vi "PMTreadgraph.vi"(8 "error in":errorcluster, 10 "queue in":refnum<queue>, 11 "PMT chart":refnum<vi>) -> (0 "error out":errorcluster)   [LabVIEW 2019]
uses:
  <vilib>/Analysis/baseanly.llb/Mean (DBL).vi
  <vilib>/Utility/error.llb/Error Cluster From Error Code.vi
  <vilib>/rvi/errors/niLvFpgaAdjustHostInterfaceError.vi
  GlobalImagingStatus.vi
  <vilib>/rvi/interface/nirviReadWriteControl/nirviReadWriteControl.xnode
  <vilib>/Analysis/NI_AALBase.lvlib
  Global.lvlib
  NiFpgaLv.dll
  <vilib>/rvi/interface/Simulation/niFpgaSimulationCallBeginRW.vi
panel:
  out "PMT saturation 2":bool
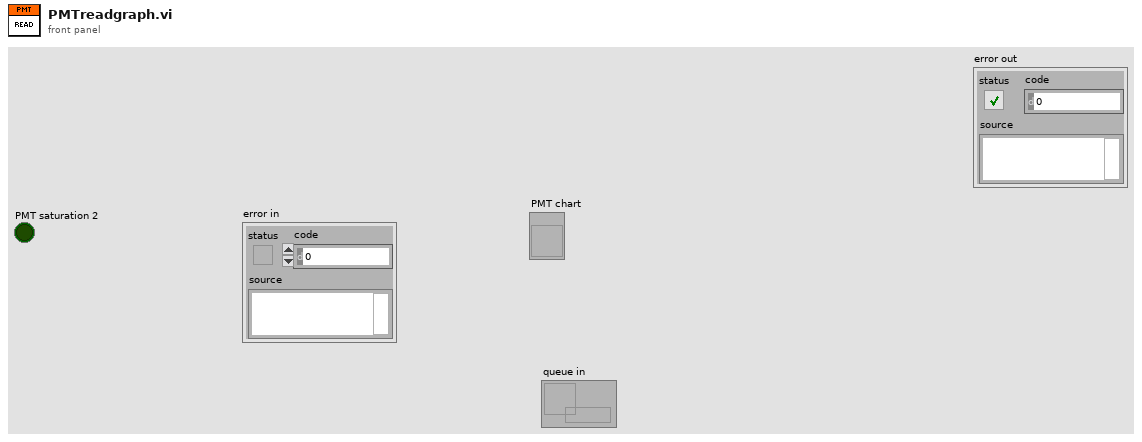
[diagram p1: front panel]
types:
  T1 = typedef "ImagingStatusControl.ctl" = enum16{"PMT_large", "Camera_large", "PMT", "Camera", "Idle"}
  T2 = cluster{"Frequency Chart":u32, "Frequency Chart":u32}
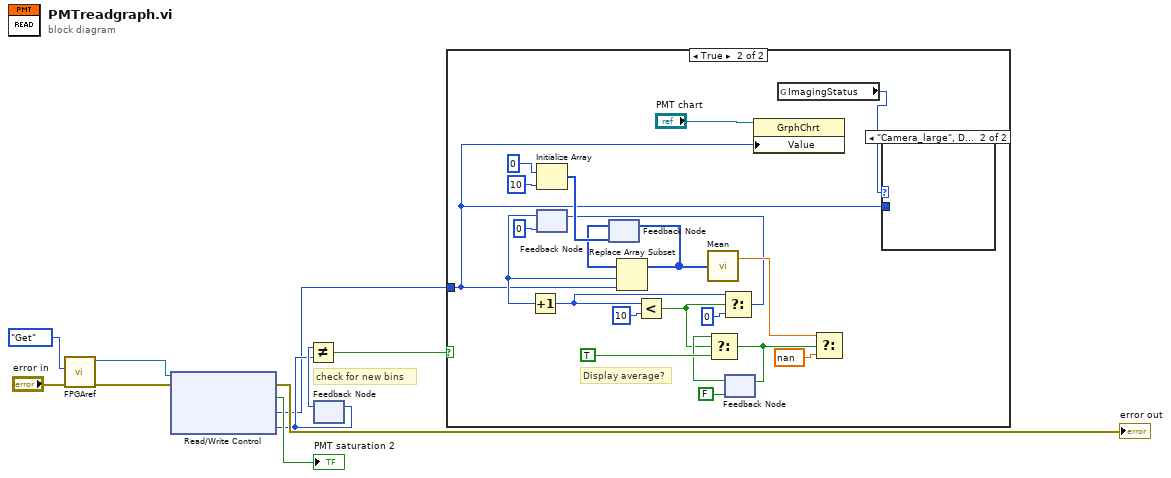
[diagram p0: block diagram]
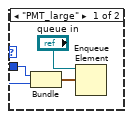
[diagram p3: hidden frame]
diagram:
  # "check for new bins"
  n1 = call "FPGAref.vi"("error in"="error in", "Enum"=enum16{"Set", "Get"}."Get") -> ("error out"=w7:errorcluster, "FPGA VI Reference Out 2"=w8:refnum<k20>)  [unwired: 4 in]
  n2 = xnode "Read/Write Control"("FPGA VI Reference In"=w8, "error in"=w7) -> ("error out"=→"error out":errorcluster, "PMT saturation"=→"PMT saturation 2":bool, "Frequency Chart"=w1:u32, "bin number"=w3:u32)  [unwired: 1 out]
  n3 = feedback #1() -> (w4:u32)  [unwired: 1 in]
  n4 = Not Equal?(x=w4, y=w3) -> (x != y?=w2:bool)
  n5 = feedback-in #1(w3) -> ()
  n6 = case shown="True" w2 {
    tunnel: w1 -> [_ w12]
    frame False {
    }
    frame True {
      # "Display average?"
      n7 = Initialize Array(u32 0 ("Frequency Chart"), 10 ("dimension size")) -> (w29:u32[])
      n8 = feedback #2(0) -> (w23:i32)
      n9 = Increment(x=w23) -> (x+1=w20:i32)
      n10 = feedback #3(w29) -> (w28:u32[])
      n11 = Replace Array Subset(array=w28, new element=w12, index=w23) -> (w27:u32[])
      n12 = feedback-in #3(w27) -> ()
      n13 = Less?(x=w20, y=10) -> (x < y?=w15:bool)
      n14 = call-poly <vilib>:"Mean.vi"("X"=w27) -> ("mean"=w26:dbl)  [unwired: 1 out]
      n15 = Select(t=w20, s=w15, f=0) -> (s? t:f=w19:i32)
      n16 = feedback-in #2(w19) -> ()
      n17 = feedback #4(FALSE) -> (w16:bool)
      n18 = Select(t=w16, s=w15, f=TRUE) -> (s? t:f=w14:bool)
      n19 = feedback-in #4(w14) -> ()
      n20 = property class="GrphChrt"(reference="PMT chart", "Value"=w12) -> ()  [unwired: 1 in, 2 out]
      n21 = global read "GlobalImagingStatus.vi" "ImagingStatus"() -> (w11:T1)
      n22 = Select(t=w26, s=w14, f=nan) -> ()  [unwired: 1 out]
      n23 = case shown="\"Camera_large\", Default" w11 {
        tunnel: w12 -> [w33 _]
        frame "PMT_large" {
          n24 = Bundle("Frequency Chart"=w33, "Frequency Chart"=w33) -> (w32:T2)  [unwired: 1 in]
          n25 = Enqueue Element(queue="queue in", element=w32) -> ()  [unwired: 2 in, 3 out]
        }
        frame "Camera_large", Default {
        }
      }
    }
  }
